vi "Global List.vi"(8 "error in (no error)":errorcluster, 11 "Global in":refnum<k1>) -> (0 "error out":errorcluster, 2 "Instances":T1[](array[typedef]), 3 "Global out":refnum<k1>)   [LabVIEW 2018, in "Shared.lvlib"]
uses:
  Shared.lvlib
  Controls/Global.ctl
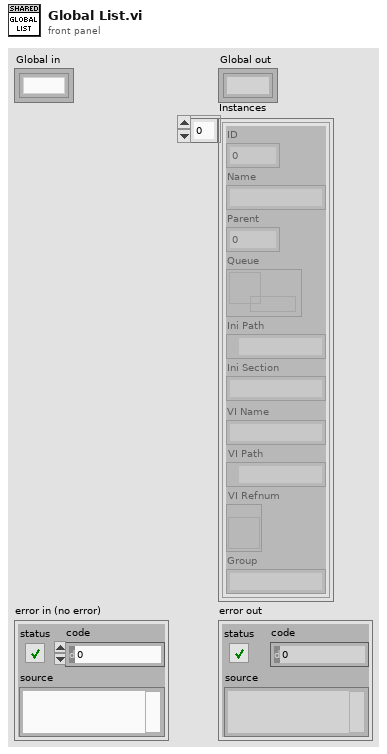
[diagram p1: front panel]
types:
  T1 = typedef "Shared.lvlib/Global.ctl" = cluster{"ID":i32, "Name":string, "Parent":i32, "Queue":refnum<queue>, "Ini Path":path, "Ini Section":string, "VI Name":string, "VI Path":path, "VI Refnum":refnum<vi>, "Group":string}
  T2 = cluster{"ID":i32, "Name":string, "Parent":i32, "Queue":refnum<queue>, "Ini Path":path, "Ini Section":string, "VI Name":string, "VI Path":path, "VI Refnum":refnum<vi>, "Group":string}[]
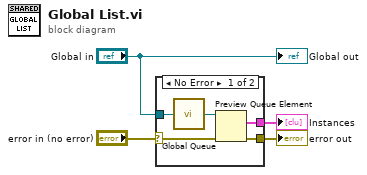
[diagram p0: block diagram]
diagram:
  n1 = case shown="No Error" "error in (no error)" {
    selector: "error in (no error)" -> [w8 w10]
    tunnel: "Global in" -> [w6 _]
    tunnel: [w9 _] -> w3
    tunnel: [w7 w10] -> w1
    frame No Error {
      n2 = call "Global Queue.vi"("Global in"=w6) -> ("Global"=w5:refnum<queue>)
      n3 = Preview Queue Element(queue=w5, error in (no error)=w8) -> (element=w9:T2, error out=w7:errorcluster)  [unwired: 1 in, 2 out]
    }
    frame Error {
    }
  }
  "error out" <- w1
  "Instances" <- w3
  "Global out" <- "Global in"
